vi "Data Type.vi"(8 "error in (no error)":errorcluster, 11 "Control in":refnum<class "Control.lvclass">) -> (0 "error out":errorcluster, 2 "Control Data Type":T1, 3 "Control out":refnum<class "Control.lvclass">)   [LabVIEW 2020, in "Aether Engine.lvlib" / "Control.lvclass"]
uses:
  Control.lvclass
  Control Data Type.ctl
  Aether Engine.lvlib
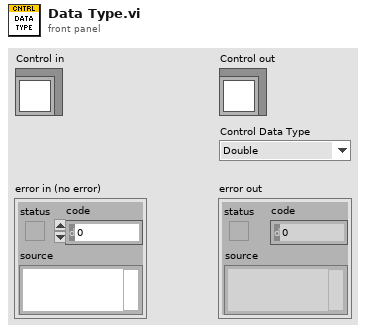
[diagram p1: front panel]
types:
  T1 = typedef "Aether Engine.lvlib/Control Data Type.ctl" = enum16{"Double", "Bool", "Chart"}
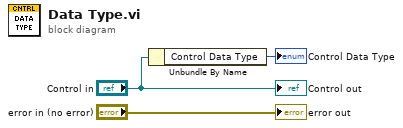
[diagram p0: block diagram]
diagram:
  n1 = Unbundle By Name("Control in") -> ("Control Data Type"=→"Control Data Type":T1)
  "error out" <- "error in (no error)"
  "Control out" <- "Control in"
